vi "Autocycle v0.5.vi"(7 "Message Queue":refnum<queue>, 8 "error in":errorcluster, 10 "All Para":cluster{"Auto Para":T1, "General Para":T2}={"Auto Para"={"Agitator Delays"=[], "TF Delays"=[], "Insertion Delays"=[], "Cutting Delays"=[], "PF Delays"=[], "Measur. Delays"=[], "Reject Delays"=[1000], "BF Delays"=[1000]}, "General Para"={"Max. Cons."=5.0, "Offset 1"=0.0, "Offset 2"=0.0, "Offset 3"=0.0, "Offset 4"=0.0, "OutputPause"=0.0, "RejectPause"=0.0}}) -> (0 "error out":errorcluster)   [LabVIEW 2017]
doc: "v0.3:\n- Added End Cycle & Stop initiated as different stops\n- Make PF & TF not run on the first iteration"
uses:
  support/Message Queue/Message Cluster.ctl
  Controls/Auto Delays.ctl
  support/Controls/General Para.ctl
  Controls/Auto Times.ctl
  Global Variables/RT GV.vi
  Global Variables/FPGA GV.vi
  <vilib>/Utility/error.llb/Error Cluster From Error Code.vi
  <vilib>/rvi/errors/niLvFpgaAdjustHostInterfaceError.vi
  support/Message Queue/Enqueue Message (Single).vi
  <vilib>/rvi/interface/nirviReadWriteControl/nirviReadWriteControl.xnode
  Controls/FPGA Ref.ctl
  NiFpgaLv.dll
  <vilib>/rvi/interface/Simulation/niFpgaSimulationCallBeginRW.vi
  support/Message Queue/Message Queue.lvlib
panel:
  in  "EnableSOL":bool=TRUE
  out "Iterations to ON":i32
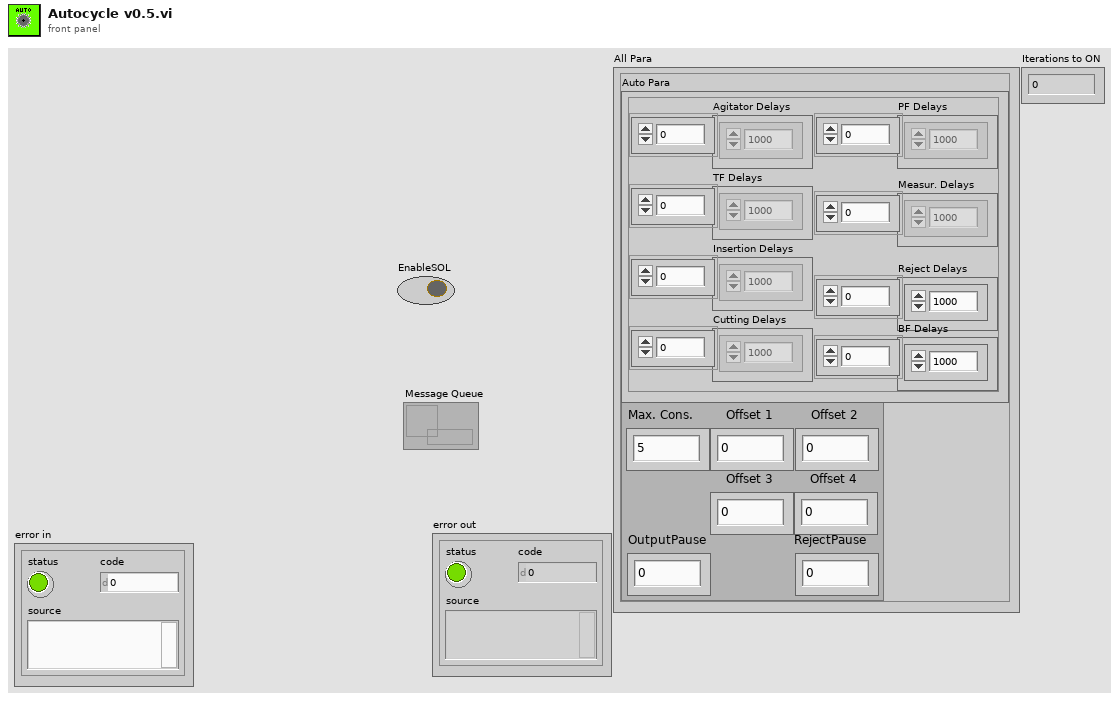
[diagram p1: front panel]
types:
  T1 = typedef "Auto Delays.ctl" = cluster{"Agitator Delays":u32[], "TF Delays":u32[], "Insertion Delays":u32[], "Cutting Delays":u32[], "PF Delays":u32[], "Measur. Delays":dbl[], "Reject Delays":u32[], "BF Delays":u32[]}
  T2 = typedef "General Para.ctl" = cluster{"Max. Cons.":dbl, "Offset 1":dbl, "Offset 2":dbl, "Offset 3":dbl, "Offset 4":dbl, "OutputPause":dbl, "RejectPause":dbl}
  T3 = typedef "FPGA Ref.ctl" = refnum<k20>
  T4 = cluster{"TL_Red":bool, "TL_Orange":bool, "TL_Green":bool, "TL_Buzzer":bool, "SOL_Index_Rotary_CW":bool, "SOL_Index_CNVR_Rotary_CCW":bool, "SOL_Index_CNVR_Stopper_Rear":bool, "SOL_Index_CNVR_Output _Separator _Rear":bool, "Bowl Feeder_ ON1":bool, "Pump_CNVR_Motor _ON":bool, "SOL_PC_Gating_CYL_Rear":bool, "SOL_Tube_Feed_Agitatator":bool, "SOL_Tube_Feed_Gating_CYL":bool, "SOL_Insertion _CYL":bool, "SOL_Insertion_Clamp_CYL":bool, "SOL_Cutting_CYL":bool, "SOL_Cutting_Clamp_CYL":bool, "SOL_Insertion_Air_Nozzle":bool, "SOL_Measurement_CYL":bool, "DO1.19":bool, "SOL_Rejection CYL_1":bool, "SOL_Rejection CYL_2":bool, "SOL_Rejection CYL_3":bool, "SOL_Rejection CYL_4":bool, "Bowl Feeder_ON2":bool, "SOL_BF_BlowerON":bool, "SOL_BF1_Track1":bool, "SOL_BF1_Track2":bool, "SOL_BF2_Track1":bool, "SOL_BF2_Track2":bool, "DO1.30":bool, "DO1.31":bool}
  T5 = typedef "Auto Times.ctl" = cluster{"Index Time":u32, "TF Time":u32, "Insertion Time":u32, "Cutting Time":u32, "PF Time":u32, "Meas. Time":u32, "Reject Time":u32}
  T6 = cluster{"Reject 1":bool, "Reject 2":bool, "Reject 3":bool, "Reject 4":bool}
  T7 = cluster{"Tube Present":bool[], "Parts Count":u32}
  T8 = cluster{"seconds since 1Jan1904":timestamp, "Auto Times":T5, "Tube Present":bool[], "Reject Pallets":cluster{"Reject 1":bool, "Reject 2":bool, "Reject 3":bool, "Reject 4":bool}, "Measurements":cluster{"1":dbl, "2":dbl, "3":dbl, "4":dbl}}
  T9 = typedef "Auto Stats.ctl" = cluster{"Time-Stamp":timestamp, "Auto Times":T5, "Measurements":cluster{"1":dbl, "2":dbl, "3":dbl, "4":dbl}, "Outputs":cluster{"Good Parts":u32, "Reject Parts":u32}, "Cycle Time":dbl, "Remarks":string}
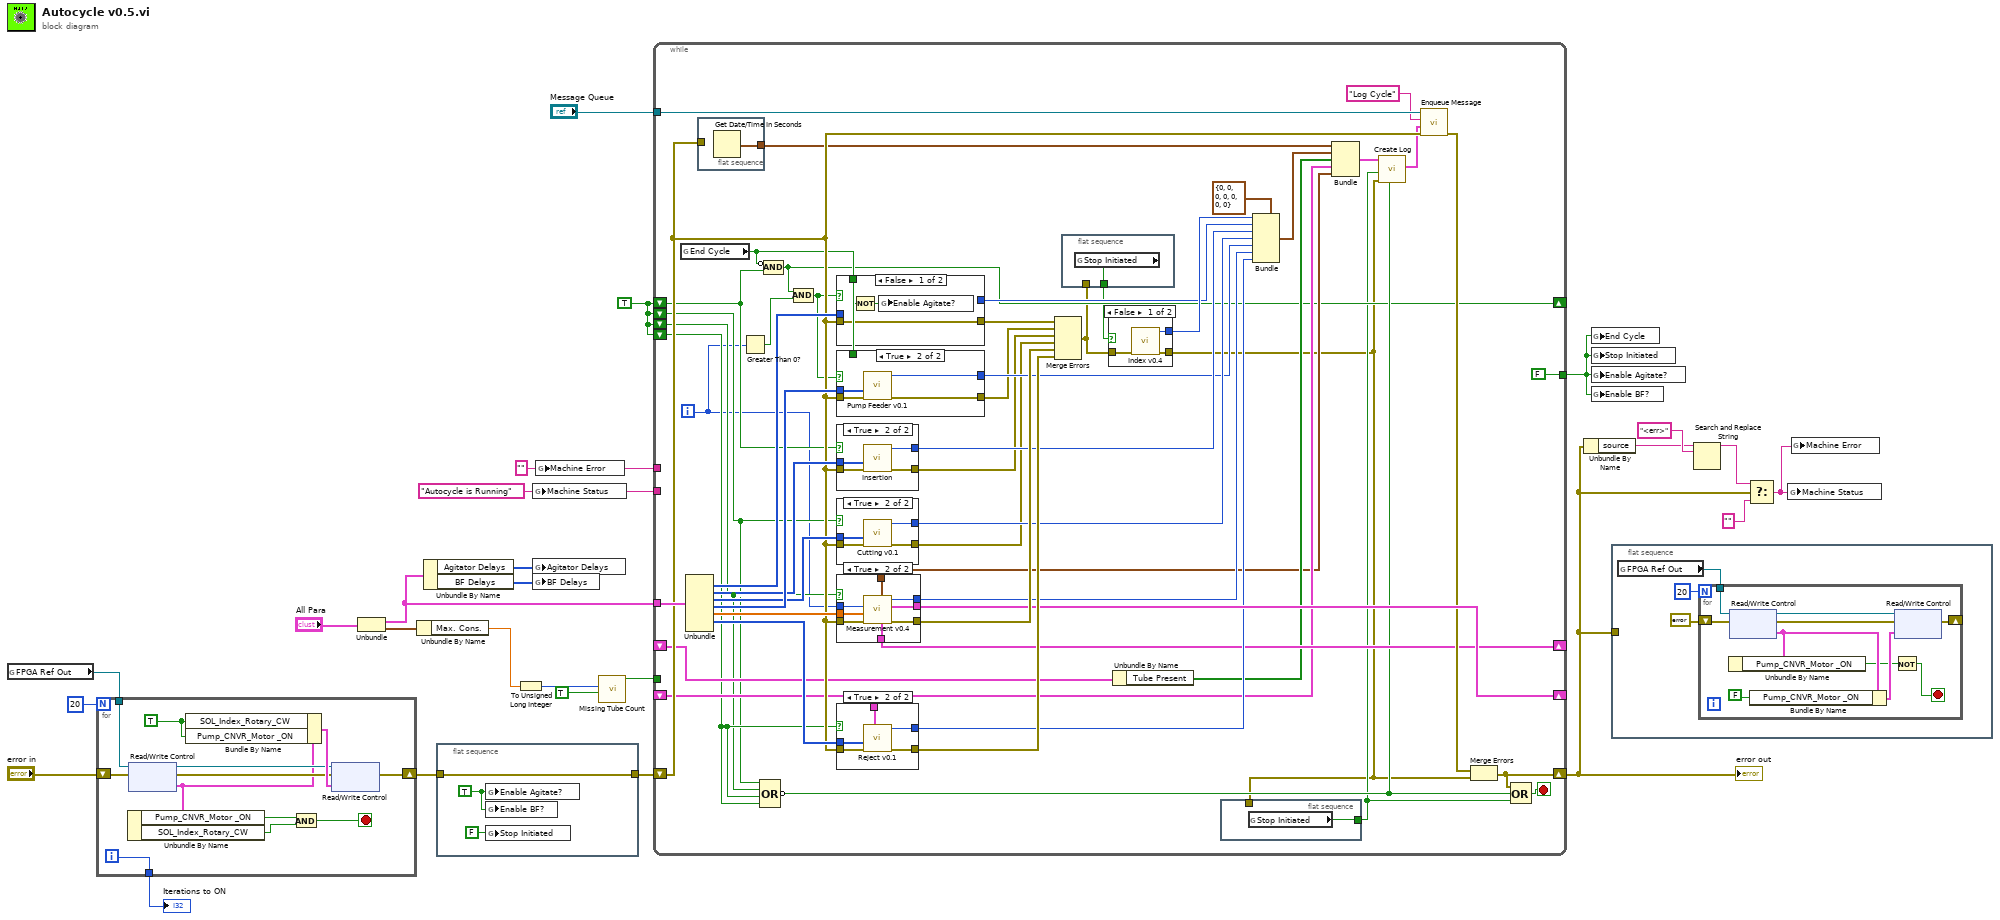
[diagram p0: block diagram]
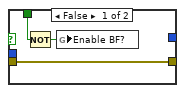
[diagram p3: hidden frame]
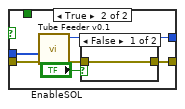
[diagram p6: hidden frame]
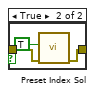
[diagram p7: hidden frame]
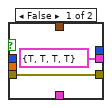
[diagram p9: hidden frame]
diagram:
  w14 = "" ("Machine Error")
  w21 = "Autocycle is Running" ("Machine Status")
  w8 = TRUE
  n1 = global read "FPGA GV.vi" "FPGA Ref Out"() -> (w24:T3)
  n2 = for {
    N: 20 -> [_]
    tunnel: w24 -> [w38]
    shift-right: [w33] -> w11
    shift-left: "error in" -> [w34]
    tunnel: [w27] -> w1
    i -> [w27]
    stop <- w29 stop-if-true
    w30 = TRUE ("Pump_CNVR_Motor _ON")
    n3 = xnode "Read/Write Control"("FPGA VI Reference In"=w38, "error in"=w34) -> ("FPGA VI Reference Out"=w35:T3, "error out"=w36:errorcluster, "DO 1"=w32:T4)
    n4 = Unbundle By Name(w32) -> ("Pump_CNVR_Motor _ON"=w31:bool, "SOL_Index_Rotary_CW"=w28:bool)
    n5 = Bundle By Name(cluster=w32, "SOL_Index_Rotary_CW"=w30, "Pump_CNVR_Motor _ON"=w30) -> (w37:T4)
    n6 = Compound Arithmetic op=AND(w31, w28) -> (w29:bool)
    n7 = xnode "Read/Write Control"("FPGA VI Reference In"=w35, "error in"=w36, "DO 1"=w37) -> ("error out"=w33:errorcluster)  [unwired: 1 out]
  }
  "Iterations to ON" <- w1
  n8 = Unbundle("All Para") -> ("Auto Para"=w5:T1, "General Para"=w4:T2)
  n9 = Unbundle By Name(w4) -> ("Max. Cons."=w3:dbl)
  n10 = Unbundle By Name(w5) -> ("Agitator Delays"=w26:u32[], "BF Delays"=w25:u32[])
  n11 = flat-sequence {
    tunnel: [w41] -> w10
    tunnel: w11 -> [w41]
    frame #0 {
      w40 = TRUE ("Enable Agitate?")
      n12 = global write "RT GV.vi" "Enable Agitate?"(w40) -> ()
      n13 = global write "RT GV.vi" "Enable BF?"(w40) -> ()
      n14 = global write "RT GV.vi" "Stop Initiated"(FALSE ("Stop Initiated")) -> ()
    }
  }
  n15 = To Unsigned Long Integer(number=w3) -> (unsigned 32bit integer=w2:u32)
  n16 = global write "RT GV.vi" "Machine Status"(w21) -> ()
  n17 = global write "RT GV.vi" "Agitator Delays"(w26) -> ()
  n18 = global write "RT GV.vi" "BF Delays"(w25) -> ()
  n19 = global write "RT GV.vi" "Machine Error"(w14) -> ()
  n20 = call "Missing Tube Count.vi"("ResetMT?"=TRUE, "Max Successive"=w2) -> ("Boolean"=w12:bool)  [unwired: 8 in, 1 out]
  n21 = while {
    tunnel: w5 -> [w89]
    shift-right: [w66] -> w19
    shift-left: w10 -> [w67]
    shift-right: [w83] -> _
    shift-left: _ -> [w58]
    shift-right: [w49] -> _
    shift-left: w8 -> [w50]
    shift-left: w8 -> [w51]
    shift-left: w8 -> [w52]
    shift-left: w8 -> [w53]
    tunnel: "Message Queue" -> [w73]
    tunnel: [FALSE] -> w7
    tunnel: w21 -> [_]
    tunnel: w14 -> [_]
    shift-right: [w61] -> _
    shift-left: _ -> [w60]
    tunnel: w12 -> [_]
    i -> [w45]
    stop <- w82 stop-if-true
    n22 = global read "RT GV.vi" "End Cycle"() -> (w54:bool)
    n23 = Unbundle(w89) -> ("TF Delays"=w92:u32[], "Insertion Delays"=w91:u32[], "Cutting Delays"=w90:u32[], "PF Delays"=w93:u32[], "Measur. Delays"=w87:dbl[], "Reject Delays"=w85:u32[])  [unwired: 2 out]
    n24 = flat-sequence {
      tunnel: w67 -> [_]
      tunnel: [w100] -> w63
      frame #0 {
        n25 = Get Date/Time In Seconds() -> (seconds since 1Jan1904=w100:timestamp)
      }
    }
    n26 = Greater Than 0?(x=w45) -> (x > 0?=w47:bool)
    n27 = Compound Arithmetic op=OR(w51, w52, w53, w53) -> (invert w56:bool)
    n28 = Compound Arithmetic op=AND(invert w54, w50) -> (w49:bool)
    n29 = Compound Arithmetic op=AND(w49, w47) -> (w48:bool)
    n30 = case shown="False" w48 {
      tunnel: w67 -> [w120 w126]
      tunnel: [w120 w122] -> w88
      tunnel: w92 -> [_ w125]
      tunnel: [_ w124] -> w80
      tunnel: w54 -> [w119 _]
      frame False {
        n31 = Not(x=w119) -> (.not. x?=w118:bool)
        n32 = global write "RT GV.vi" "Enable Agitate?"(w118) -> ()
      }
      frame True {
        n33 = call "Tube Feeder v0.1.vi"("error in (no error)"=w126, "TF Para"=w125) -> ("error out"=w123:errorcluster, "TF Time"=w124:u32)  [unwired: 8 in]
        n34 = case shown="False" "EnableSOL" {
          tunnel: w123 -> [w127 w130]
          tunnel: [w127 w129] -> w122
          frame False {
          }
          frame True {
            n35 = call "Preset Index Sol.vi"("error in"=w130, "CCW?"=TRUE) -> ("error out"=w129:errorcluster)  [unwired: 9 in]
          }
        }
      }
    }
    n36 = case shown="True" w48 {
      tunnel: w67 -> [w103 w107]
      tunnel: [w103 w106] -> w69
      tunnel: w93 -> [_ w105]
      tunnel: [_ w104] -> w77
      tunnel: w54 -> [w102 _]
      frame False {
        n37 = Not(x=w102) -> (.not. x?=w101:bool)
        n38 = global write "RT GV.vi" "Enable BF?"(w101) -> ()
      }
      frame True {
        n39 = call "Pump Feeder v0.1.vi"("error in (no error)"=w107, "TF Delays"=w105) -> ("error out"=w106:errorcluster, "PF Time"=w104:u32)  [unwired: 8 in]
      }
    }
    n40 = case shown="True" w50 {
      tunnel: w67 -> [w113 w117]
      tunnel: [w113 w116] -> w70
      tunnel: w91 -> [_ w115]
      tunnel: [_ w114] -> w79
      frame False {
      }
      frame True {
        n41 = call "Insertion.vi"("error in (no error)"=w117, "Insertion Delays"=w115) -> ("error out"=w116:errorcluster, "Insertion Time"=w114:u32)  [unwired: 7 in, 1 out]
      }
    }
    n42 = case shown="True" w51 {
      tunnel: w67 -> [w108 w112]
      tunnel: [w108 w111] -> w71
      tunnel: w90 -> [_ w110]
      tunnel: [_ w109] -> w78
      frame False {
      }
      frame True {
        n43 = call "Cutting v0.1.vi"("error in (no error)"=w112, "Cutting Delays"=w110) -> ("error out"=w111:errorcluster, "Cutting Time"=w109:u32)  [unwired: 8 in]
      }
    }
    n44 = case shown="True" w52 {
      tunnel: w67 -> [w138 w146]
      tunnel: [w138 w145] -> w86
      tunnel: w87 -> [_ w144]
      tunnel: [_ w143] -> w76
      tunnel: [_ w142] -> w57
      tunnel: [T6 {"Reject 1"=TRUE, "Reject 2"=TRUE, "Reject 3"=TRUE, "Reject 4"=TRUE} ("Reject Pallets") w141] -> w83
      tunnel: [_ w140] -> w61
      tunnel: w45 -> [_ w139]
      frame False {
      }
      frame True {
        n45 = call "Measurement v0.4.vi"("error in (no error)"=w146, "TF Delays"=w144, "Loop Count"=w139) -> ("error out"=w145:errorcluster, "Reject Pallets"=w141:T6, "PF Time"=w143:u32, "Part Count"=w140:T7, "Measurements"=w142:cluster{"1":dbl, "2":dbl, "3":dbl, "4":dbl})  [unwired: 4 in]
      }
    }
    n46 = case shown="True" w53 {
      tunnel: w67 -> [w131 w136]
      tunnel: [w131 w135] -> w84
      tunnel: w85 -> [_ w134]
      tunnel: [_ w133] -> w75
      tunnel: w58 -> [_ w132]
      frame False {
      }
      frame True {
        n47 = call "Reject v0.1.vi"("Reject Pallets"=w132, "error in (no error)"=w136, "TF Delays"=w134) -> ("error out"=w135:errorcluster, "PF Time"=w133:u32)  [unwired: 7 in]
      }
    }
    n48 = Merge Errors(w88, w69, w70, w71, w86, w84) -> (w42:errorcluster)
    n49 = flat-sequence {
      tunnel: [w94] -> w43
      tunnel: w42 -> [_]
      frame #0 {
        n50 = global read "RT GV.vi" "Stop Initiated"() -> (w94:bool)
      }
    }
    n51 = case shown="False" w43 {
      tunnel: [w97 _] -> w81
      tunnel: w42 -> [w96 w98]
      tunnel: [w95 w98] -> w44
      frame False {
        n52 = call "Index v0.4.vi"("error in (no error)"=w96) -> ("error out"=w95:errorcluster, "Index Time"=w97:u32)  [unwired: 7 in, 2 out]
      }
      frame True {
      }
    }
    n53 = Unbundle By Name(w60) -> ("Tube Present"=w59:bool[])
    n54 = flat-sequence {
      tunnel: [w99] -> w46
      tunnel: w44 -> [_]
      frame #0 {
        n55 = global read "RT GV.vi" "Stop Initiated"() -> (w99:bool)
      }
    }
    n56 = Bundle(cluster=T5 {"Index Time"=0, "TF Time"=0, "Insertion Time"=0, "Cutting Time"=0, "PF Time"=0, "Meas. Time"=0, "Reject Time"=0} ("Auto Times"), "Index Time"=w81, "TF Time"=w80, "Insertion Time"=w79, "Cutting Time"=w78, "PF Time"=w77, "Meas. Time"=w76, "Reject Time"=w75) -> (w62:T5)
    n57 = Bundle("seconds since 1Jan1904"=w63, "Auto Times"=w62, "Tube Present"=w59, "Reject Pallets"=w58, "Measurements"=w57) -> (w55:T8)  [unwired: 1 in]
    n58 = call "Create Log.vi"("End Cycle?"=w56, "Error in"=w44, "Stop Initiated?"=w46, "Log Input Data"=w55) -> ("Auto Stats"=w64:T9)  [unwired: 7 in]
    n59 = call-poly "Enqueue Message.vi"("error in (no error)"=w67, "Message Data"=w64, "Message"="Log Cycle", "Message Queue"=w73) -> ("error out"=w65:errorcluster)  [unwired: 6 in, 1 out]
    n60 = Merge Errors(w65, w44) -> (w66:errorcluster)
    n61 = Compound Arithmetic op=OR(w66, w56, w46) -> (w82:bool)
  }
  "error out" <- w19
  n62 = Unbundle By Name(w19) -> ("source"=w17:string)
  n63 = global write "RT GV.vi" "End Cycle"(w7) -> ()
  n64 = global write "RT GV.vi" "Stop Initiated"(w7) -> ()
  n65 = global write "RT GV.vi" "Enable Agitate?"(w7) -> ()
  n66 = global write "RT GV.vi" "Enable BF?"(w7) -> ()
  n67 = flat-sequence {
    tunnel: w19 -> [_]
    frame #0 {
      n68 = global read "FPGA GV.vi" "FPGA Ref Out"() -> (w148:T3)
      n69 = for {
        N: 20 -> [_]
        tunnel: w148 -> [w159]
        shift-right: [w153] -> _
        shift-left: errorcluster {"status"=FALSE, "code"=0, "source"=""} ("error out") -> [w154]
        stop <- w150 stop-if-true
        n70 = xnode "Read/Write Control"("FPGA VI Reference In"=w159, "error in"=w154) -> ("FPGA VI Reference Out"=w155:T3, "error out"=w156:errorcluster, "DO 1"=w152:T4)
        n71 = Unbundle By Name(w152) -> ("Pump_CNVR_Motor _ON"=w151:bool)
        n72 = Bundle By Name(cluster=w152, "Pump_CNVR_Motor _ON"=FALSE) -> (w158:T4)
        n73 = Not(x=w151) -> (.not. x?=w150:bool)
        n74 = xnode "Read/Write Control"("FPGA VI Reference In"=w155, "error in"=w156, "DO 1"=w158) -> ("error out"=w153:errorcluster)  [unwired: 1 out]
      }
    }
  }
  n75 = Search and Replace String(input string=w17, search string="<err>") -> (result string=w16:string)  [unwired: 6 in, 3 out]
  n76 = Select(t=w16, s=w19, f="" ("Machine Status")) -> (s? t:f=w15:string)
  n77 = global write "RT GV.vi" "Machine Status"(w15) -> ()
  n78 = global write "RT GV.vi" "Machine Error"(w15) -> ()
